vi "How to use in host.vi"(9 "element":string) -> (1 "2D Picture":picture, 11 "Select Part":u16(ring) items=["P1.JPG", "P10.JPG", "P11.JPG", "P13.JPG", "P14.JPG", "P2.JPG", "P3.JPG", "P4.JPG", "P5.JPG", "P6.JPG", "P7.JPG", "P8.jpg"])   [LabVIEW 2015]
uses:
  Galobal variable_TI.vi
panel:
  out "error out":errorcluster
  out "empty?":bool
  in  "stop":bool
  out "filenames":string[](array[string])
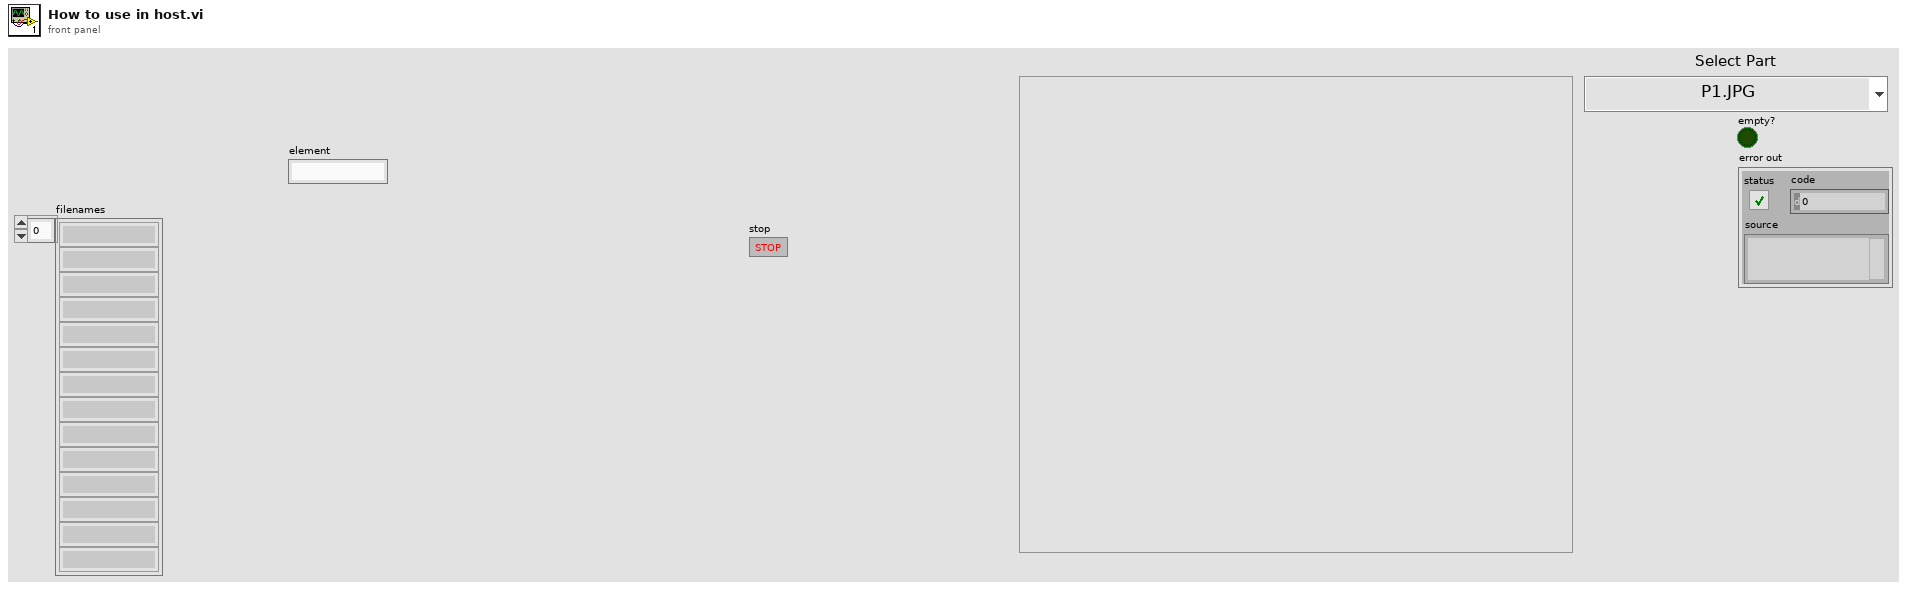
[diagram p1: front panel]
types:
  T1 = typedef "imagedata.ctl" = cluster{"image type":i32, "image depth":i32, "image":u8[], "mask":u8[], "colors":u32[], "Rectangle":cluster{"left":i16, "top":i16, "right":i16, "bottom":i16}}
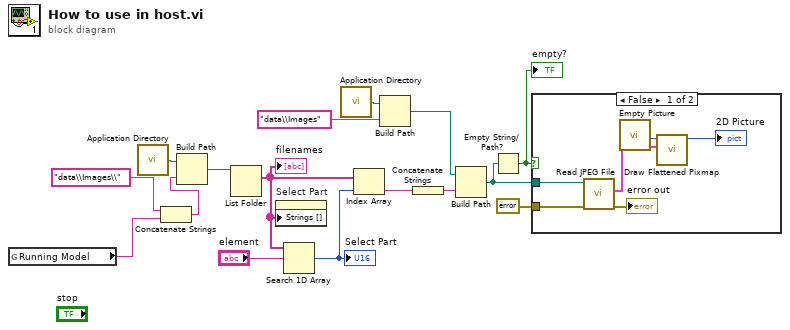
[diagram p0: block diagram]
diagram:
  n1 = global read "Galobal variable_TI.vi" "Running Model"() -> (w2:string)
  n2 = call <vilib>:"Application Directory.vi"() -> ("Application Directory"=w16:path)
  n3 = Concatenate Strings("data\\Images\\" ("name or relative path"), w2) -> (w1:string)
  n4 = Build Path(base path=w16, name or relative path=w1) -> (appended path=w15:path)
  n5 = List Folder(path=w15) -> (filenames=w14:string[])  [unwired: 3 in, 3 out]
  "filenames" <- w14
  n6 = property on="Select Part" class="Ring (strict)"("Strings []"=w14) -> ()  [unwired: 2 in, 2 out]
  n7 = Search 1D Array(1D array=w14, element="element") -> (index of element=w13:i32)  [unwired: 1 in]
  "Select Part" <- w13
  n8 = call <vilib>:"Application Directory.vi"() -> ("Application Directory"=w10:path)
  n9 = Index Array(array=w14, index=w13) -> (element=w7:string)
  n10 = Build Path(base path=w10, name or relative path="data\\Images") -> (appended path=w8:path)
  n11 = Concatenate Strings(w7) -> (w11:string)
  n12 = Build Path(base path=w8, name or relative path=w11) -> (appended path=w6:path)
  n13 = Empty String/Path?(string/path=w6) -> (empty?=w5:bool)
  "empty?" <- w5
  n14 = case shown="False" w5 {
    tunnel: w6 -> [w19 _]
    tunnel: errorcluster {"status"=FALSE, "code"=0, "source"=""} ("error in (no error)") -> [w18 _]
    frame False {
      n15 = call <vilib>:"Read JPEG File.vi"("error in (no error)"=w18, "path to JPEG file"=w19) -> ("error out"=→"error out":errorcluster, "image data"=w21:T1)  [unwired: 7 in, 1 out]
      n16 = call "Empty Picture"() -> ("empty picture"=w22:picture)
      n17 = call <vilib>:"Draw Flattened Pixmap.vi"("image data"=w21, "picture"=w22) -> ("new picture"=→"2D Picture":picture)  [unwired: 7 in]
    }
    frame True {
    }
  }
